vi "close.vi"(8 "error in (no error)":errorcluster, 11 "TTL_input in":refnum<class "TTL_input.lvclass">) -> (0 "error out":errorcluster, 3 "TTL_input out":refnum<class "TTL_input.lvclass">)   [LabVIEW 2013, in "TTL_input.lvclass"]
uses:
  TTL_input.lvclass
  TTL_input.lvclass/TTL_input.ctl
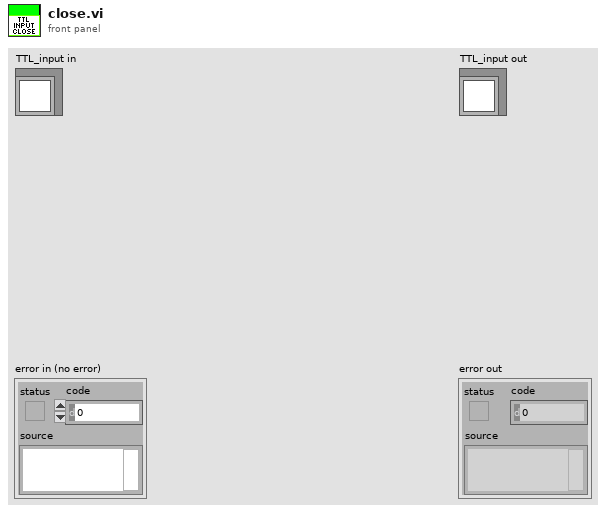
[diagram p1: front panel]
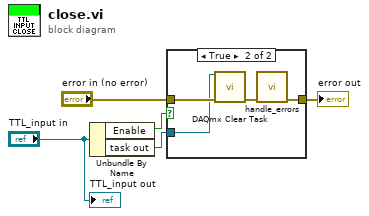
[diagram p0: block diagram]
diagram:
  n1 = Unbundle By Name("TTL_input in") -> ("Enable"=w1:bool, "task out"=w2:refnum<k21>)
  n2 = case shown="True" w1 {
    tunnel: "error in (no error)" -> [w6 w10]
    tunnel: [w6 w9] -> w4
    tunnel: w2 -> [_ w8]
    frame False {
    }
    frame True {
      n3 = call <vilib>:"DAQmx Clear Task.vi"("task in"=w8, "error in"=w10) -> ("error out"=w7:errorcluster)  [unwired: 13 in]
      n4 = call "handle_errors.vi"("error in (no error)"=w7) -> ("error out"=w9:errorcluster)  [unwired: 14 in]
    }
  }
  "error out" <- w4
  "TTL_input out" <- "TTL_input in"
